vi "About Dependency Inspector.vi"(8 "error in":errorcluster) -> (0 "error out":errorcluster)   [LabVIEW 2020, in "SimpleDependencyInspector.lvlib"]
uses:
  SimpleDependencyInspector.lvlib
  <vilib>/Platform/browser.llb/Open URL in Default Browser (string).vi
panel:
  out "Version":string
  in  "Buy Me a Coffee":bool
  in  "Documentation":bool
  in  "Linkedin":bool
  in  "Facebook":bool
  in  "Twitter":bool
  in  "Website":bool
  # "Simple Dependency Inspector"
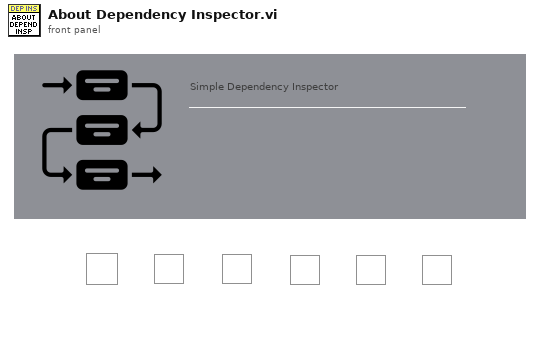
[diagram p1: front panel]
types:
  T1 = cluster{"Major":u16, "Minor":u16, "Fix":u16, "Build":u16}
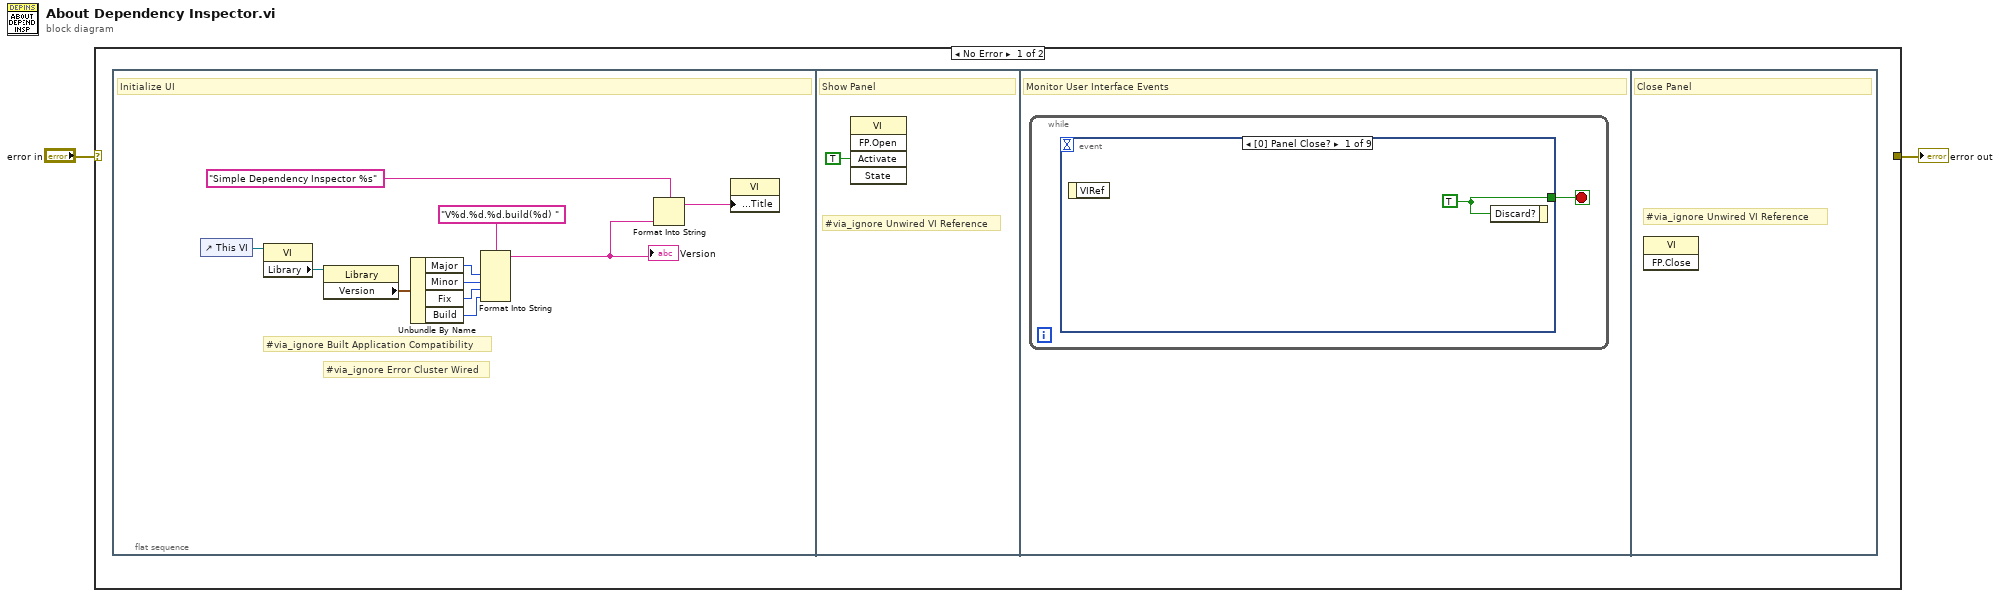
[diagram p0: block diagram]
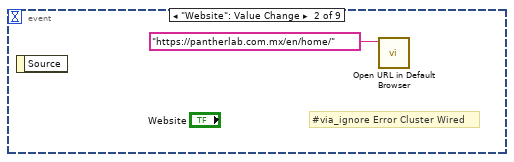
[diagram p2: hidden frame]
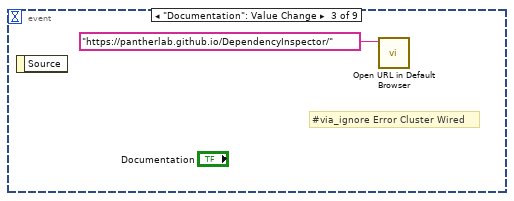
[diagram p3: hidden frame]
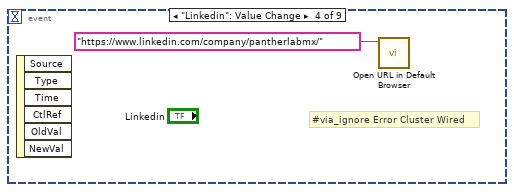
[diagram p4: hidden frame]
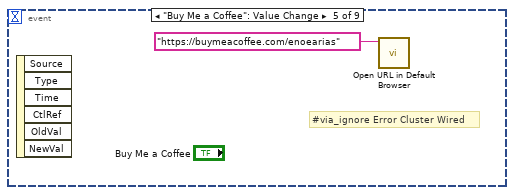
[diagram p5: hidden frame]
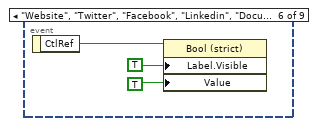
[diagram p6: hidden frame]
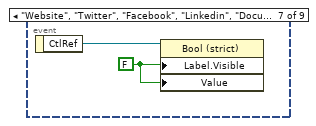
[diagram p7: hidden frame]
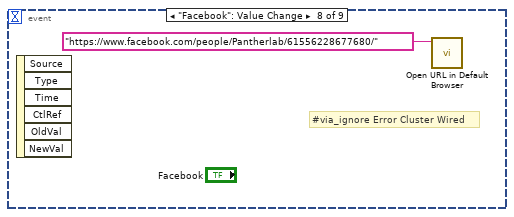
[diagram p8: hidden frame]
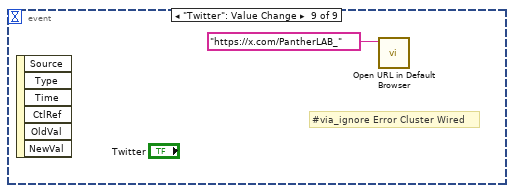
[diagram p9: hidden frame]
diagram:
  n1 = case shown="No Error" "error in" {
    selector: "error in" -> [_ w28]
    tunnel: [_ w28] -> w1
    frame No Error {
      n2 = flat-sequence {
        frame #0 {
          # "#via_ignore Built Application Compatibility"
          # "#via_ignore Error Cluster Wired"
          # "Initialize UI"
          n3 = control-ref of="This VI"() -> (w10:refnum<vi>)
          n4 = property class="VI"(reference=w10) -> ("Library"=w8:refnum<vi>)  [unwired: 1 in, 2 out]
          n5 = property class="Library"(reference=w8) -> ("Version"=w7:T1)  [unwired: 1 in, 2 out]
          n6 = Unbundle By Name(w7) -> ("Major"=w6:u16, "Minor"=w5:u16, "Fix"=w4:u16, "Build"=w3:u16)
          n7 = Format Into String(format string="V%d.%d.%d.build(%d) " ("String"), w6, w5, w4, w3) -> (resulting string=w11:string)  [unwired: 2 in, 1 out]
          "Version" <- w11
          n8 = Format Into String(format string="Simple Dependency Inspector %s" ("String"), w11) -> (resulting string=w12:string)  [unwired: 2 in, 1 out]
          n9 = property class="VI"("Front Panel.Title"=w12) -> ()  [unwired: 2 in, 2 out]
        }
        frame #1 {
          # "#via_ignore Unwired VI Reference"
          # "Show Panel"
          n10 = invoke class="VI" method="FP.Open"("Activate"=TRUE ("Activate?")) -> ()  [unwired: 4 in, 5 out]
        }
        frame #2 {
          # "Monitor User Interface Events"
          n11 = while {
            stop <- w15 stop-if-true
            n12 = event shown="[0] Panel Close?" {
              selector: _ -> [_ _ _ _ _ _ _ _ _]
              dyn-events: _ -> [_ _ _ _ _ _ _ _ _]
              timeout: _ -> [_ _ _ _ _ _ _ _ _]
              tunnel: [w16 _ _ _ _ _ _ _ _] -> w15
              event Panel Close? {
                w16 = TRUE ("Discard?")
                n13 = event-data() -> ()  [unwired: 1 in, 1 out]
                n14 = event-data("Discard?"=w16) -> ()  [unwired: 1 in, 1 out]
              }
              event "Website": Value Change {
                # "#via_ignore Error Cluster Wired"
                n15 = event-data() -> ()  [unwired: 1 in, 1 out]
                n16 = call-poly <vilib>:"Open URL in Default Browser.vi"("URL"="https://pantherlab.com.mx/en/home/") -> ()  [unwired: 5 in, 2 out]
              }
              event "Documentation": Value Change {
                # "#via_ignore Error Cluster Wired"
                n17 = event-data() -> ()  [unwired: 1 in, 1 out]
                n18 = call-poly <vilib>:"Open URL in Default Browser.vi"("URL"="https://pantherlab.github.io/DependencyInspector/") -> ()  [unwired: 5 in, 2 out]
              }
              event "Linkedin": Value Change {
                # "#via_ignore Error Cluster Wired"
                n19 = event-data() -> ()  [unwired: 1 in, 6 out]
                n20 = call-poly <vilib>:"Open URL in Default Browser.vi"("URL"="https://www.linkedin.com/company/pantherlabmx/") -> ()  [unwired: 5 in, 2 out]
              }
              event "Buy Me a Coffee": Value Change {
                # "#via_ignore Error Cluster Wired"
                n21 = event-data() -> ()  [unwired: 1 in, 6 out]
                n22 = call-poly <vilib>:"Open URL in Default Browser.vi"("URL"="https://buymeacoffee.com/enoearias") -> ()  [unwired: 5 in, 2 out]
              }
              event "Website", "Twitter", "Facebook", "Linkedin", "Documentation", "Buy Me a Coffee": Mouse Enter {
                n23 = event-data() -> ("CtlRef"=w23:refnum<vi>)  [unwired: 1 in]
                n24 = property class="Bool (strict)"(reference=w23, "Label.Visible"=TRUE, "Value"=TRUE) -> ()  [unwired: 1 in, 2 out]
              }
              event "Website", "Twitter", "Facebook", "Linkedin", "Documentation", "Buy Me a Coffee": Mouse Leave {
                w24 = FALSE ("Label.Visible")
                n25 = event-data() -> ("CtlRef"=w25:refnum<vi>)  [unwired: 1 in]
                n26 = property class="Bool (strict)"(reference=w25, "Label.Visible"=w24, "Value"=w24) -> ()  [unwired: 1 in, 2 out]
              }
              event "Facebook": Value Change {
                # "#via_ignore Error Cluster Wired"
                n27 = event-data() -> ()  [unwired: 1 in, 6 out]
                n28 = call-poly <vilib>:"Open URL in Default Browser.vi"("URL"="https://www.facebook.com/people/Pantherlab/61556228677680/") -> ()  [unwired: 5 in, 2 out]
              }
              event "Twitter": Value Change {
                # "#via_ignore Error Cluster Wired"
                n29 = event-data() -> ()  [unwired: 1 in, 6 out]
                n30 = call-poly <vilib>:"Open URL in Default Browser.vi"("URL"="https://x.com/PantherLAB_") -> ()  [unwired: 5 in, 2 out]
              }
            }
          }
        }
        frame #3 {
          # "#via_ignore Unwired VI Reference"
          # "Close Panel"
          n31 = invoke class="VI" method="FP.Close"() -> ()  [unwired: 3 in, 3 out]
        }
      }
    }
    frame Error {
    }
  }
  "error out" <- w1
